vi "AR Drone - Simple Video + Simple nav.vi"() -> ()   [LabVIEW 2014]
doc: "Very simple example showing how to use the base VIs to control the AR Drone and receive and display video data."
uses:
  Others (.ctl)/Control cluster.ctl
  <vilib>/LVH/AR Drone Toolkit/Decode NavData/Typedefs/NavData Demo.ctl
  Global.vi
  <vilib>/LVH/AR Drone Toolkit/AR Drone.lvlib
panel:
  out "Image":T1(plugin-control)
  in  "Takeoff/Land":bool
  in  "Setup Parameters":T2={"Drone IP address"="192.168.1.1", "Home IP address"="192.168.1.2", "Flight Mode"=enum."INDOOR MODE", "Mounted Hull"=enum."INDOOR HULL", "Video Camera"=2, "Max Altitude (m)"=3.0, "Max Pitch and Roll Angle (deg)"=10.0, "Max Vertical Speed (m/s)"=0.7, "Max Yaw Speed (deg/s)"=100.0} {"Video Camera" items=["Bottom Camera"=1, "Front Camera"=0, "Front in Bottom"=3, "Bottom in Front"=2]}
  in  "stop":bool
  in  "milliseconds to wait":u32=5
  out "ctr+nav":errorcluster
  out "ctr+nav":i32
  out "Battery Remaining 2":dbl(slide) scale=0.0..100.0
  out "NavData Out 2":T3
  out "Control Cluster":T4 {"Yaw Speed" scale=-1.0..1.0; "Vertical Speed" scale=-1.0..1.0; "Pitch" scale=-1.0..1.0; "Roll" scale=-1.0..1.0}
  in  "Emergency Landing":bool
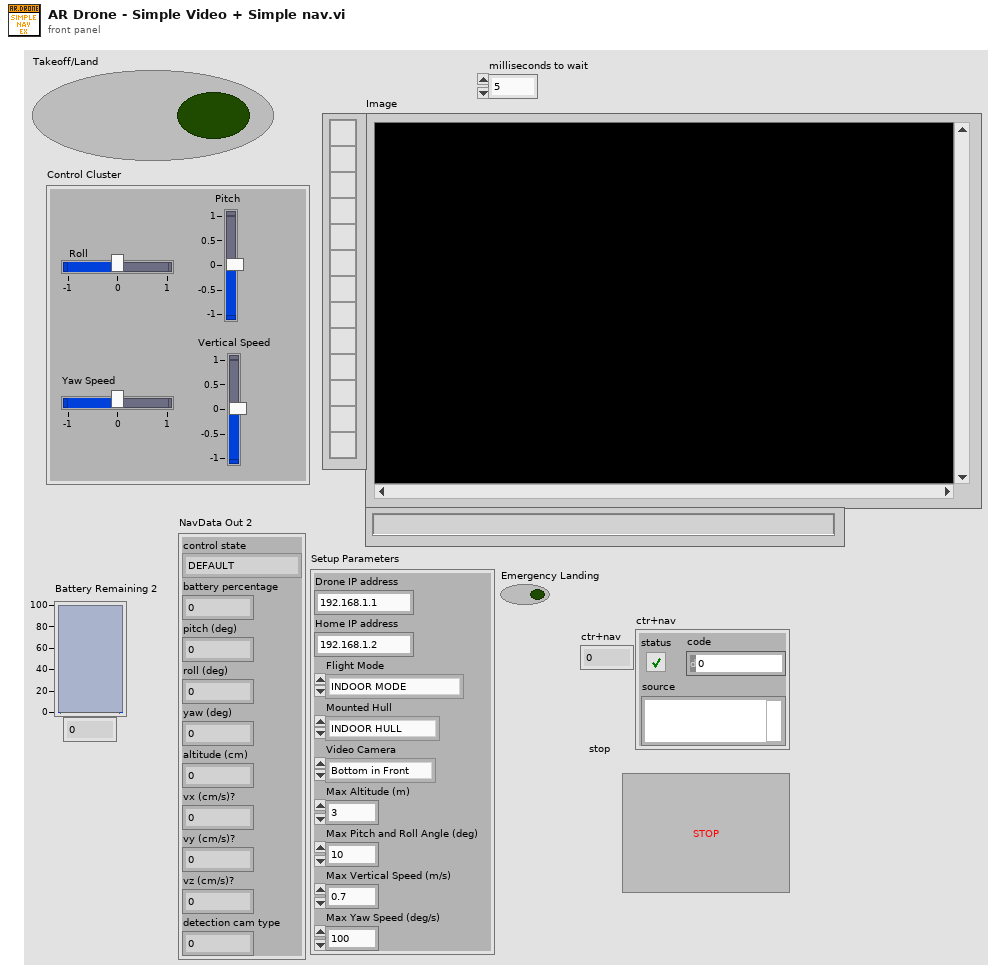
[diagram p1: front panel]
types:
  T1 = typedef "IMAQ Image.ctl" = refnum<image>
  T2 = cluster{"Drone IP address":string, "Home IP address":string, "Flight Mode":enum8{"OUTDOOR MODE", "INDOOR MODE"}, "Mounted Hull":enum8{"OUTDOOR HULL", "INDOOR HULL"}, "Video Camera":u8, "Max Altitude (m)":sgl, "Max Pitch and Roll Angle (deg)":sgl, "Max Vertical Speed (m/s)":sgl, "Max Yaw Speed (deg/s)":sgl}
  T3 = typedef "AR Drone.lvlib/NavData Demo.ctl" = cluster{"control state":enum32{"DEFAULT", "INIT", "LANDING", "FLYING", "HOVERING", "TEST", "TRANS_TAKEOFF", "TRANS_GOTOFIX", "TRANS_LANDING"}, "battery percentage":u32, "pitch (deg)":sgl, "roll (deg)":sgl, "yaw (deg)":sgl, "altitude (cm)":u32, "vx (cm/s)?":sgl, "vy (cm/s)?":sgl, "vz (cm/s)?":sgl, "detection cam type":u32}
  T4 = typedef "Control cluster.ctl" = cluster{"Roll":sgl, "Pitch":sgl, "Vertical Speed":sgl, "Yaw Speed":sgl}
  T5 = typedef "AR Drone.lvlib/AR Drone Resource.ctl" = cluster{"UDP Control Connection":refnum<k16>, "UDP NavData Connection":refnum<k16>, "UDP Video Connection (Drone 1.0)":refnum<k16>, "TCP Video Connection (Drone 2.0)":refnum<k5>, "TCP Control Port Connection":refnum<k5>, "Drone IP address":string, "Drone Command Port":u16, "Drone NavData Port":u16, "Drone Vid Stream Port":u16, "Drone TCP Control Port":u16, "Home IP address":string, "Home Command Port":u16, "Home NavData Port":u16, "Home Vid Stream Port":u16, "Drone Version":i32, "Drone Index":i32, "Command Sequence":i32}
  T6 = cluster{"button 1":bool, "button 2":bool, "button 3":bool, "button 4":bool}
  T7 = cluster{"Roll":dbl, "Pitch":dbl, "Vertical Speed":dbl, "Yaw Speed":dbl}
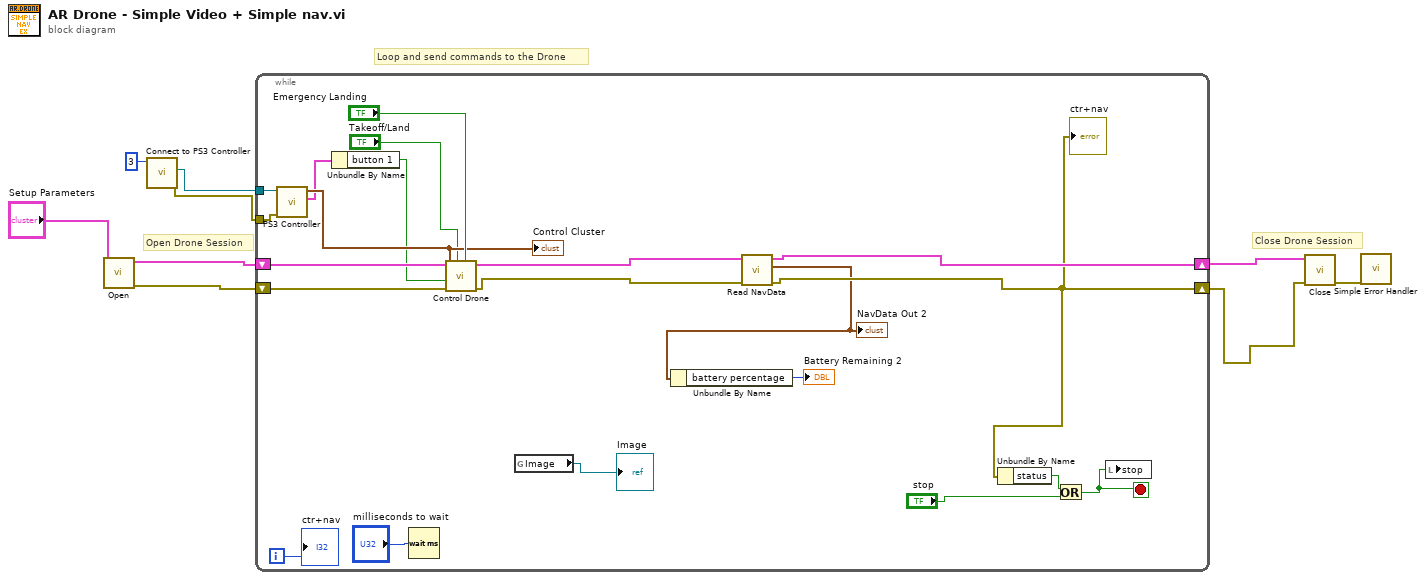
[diagram p0: block diagram]
diagram:
  # "Close Drone Session"
  # "Loop and send commands to the Drone"
  # "Open Drone Session"
  n1 = call <vilib>:"Open.vi"("Setup Parameters"="Setup Parameters") -> ("error out"=w7:errorcluster, "AR Drone Resource"=w3:T5)  [unwired: 9 in]
  n2 = call "Connect to PS3 Controller.vi"("device ID"=3) -> ("error out"=w4:errorcluster, "device ID 2"=w6:refnum<k1>)  [unwired: 7 in, 1 out]
  n3 = while {
    shift-right: [w29] -> w9
    shift-left: w3 -> [w26]
    shift-right: [w20] -> w2
    shift-left: w7 -> [w27]
    tunnel: w6 -> [w24]
    tunnel: w4 -> [w23]
    i -> [w25]
    stop <- w21 stop-if-true
    n4 = call "PS3 Controller.vi"("error in (no error)"=w23, "device ID"=w24) -> ("Buttons control"=w17:T6, "Control cluster"=w22:T7)  [unwired: 6 in, 2 out]
    "Control Cluster" <- w22
    n5 = Unbundle By Name(w17) -> ("button 1"=w16:bool)
    n6 = Wait (ms)(milliseconds to wait="milliseconds to wait") -> ()  [unwired: 1 out]
    n7 = call <vilib>:"Control Drone.vi"("Emergency Landing"="Emergency Landing", "Takeoff/Land"="Takeoff/Land", "error in (no error)"=w27, "Hover"=w16, "Control Cluster"=w22, "AR Drone Resource"=w26) -> ("error out"=w13:errorcluster, "AR Drone Resource Out"=w14:T5)  [unwired: 4 in]
    n8 = global read "Global.vi" "Image"() -> (→"Image":T1)
    n9 = call <vilib>:"Read NavData.vi"("error in (no error)"=w13, "AR Drone Resource"=w14) -> ("error out"=w20:errorcluster, "NavData Out"=w11:T3, "AR Drone Resource Out"=w29:T5)  [unwired: 7 in]
    "ctr+nav" <- w20
    "NavData Out 2" <- w11
    n10 = Unbundle By Name(w11) -> ("battery percentage"=→"Battery Remaining 2":u32)
    n11 = Unbundle By Name(w20) -> ("status"=w18:bool)
    n12 = Or(x=w18, y="stop") -> (x .or. y?=w21:bool)
    n13 = local write "stop"(w21) -> ()
    "ctr+nav" <- w25
  }
  n14 = call <vilib>:"Close.vi"("error in (no error)"=w2, "AR Drone Resource"=w9) -> ("error out"=w8:errorcluster)  [unwired: 9 in]
  n15 = call <vilib>:"Simple Error Handler.vi"("error in (no error)"=w8) -> ()  [unwired: 4 in, 5 out]
